vi "Create Base Event.vi"(9 "Event":refnum<class "Event.lvclass">, 10 "Self Event Alias":string) -> (0 "error out":errorcluster)   [LabVIEW 2021, in "jettl.lvlib"]
uses:
  jettl.lvlib
  Base Queue/Base Queue.lvlib
  Event/Event.lvclass
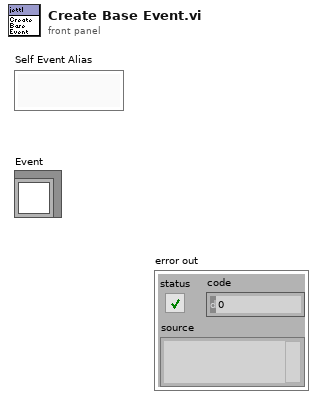
[diagram p1: front panel]
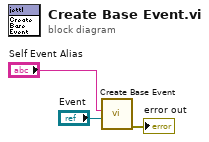
[diagram p0: block diagram]
diagram:
  n1 = call "Create Base Event.vi"("Event"="Event", "Self Event Alias"="Self Event Alias") -> ("error out"=→"error out":errorcluster)  [unwired: 9 in]
